vi "Servo Drive Test.vi"() -> ()   [LabVIEW 2019]
uses:
  LINX-PCA9865 PWM/LINX-PCA9865 PWM.lvclass
  LINX-PCA9865 PWM/LINX-PCA9865 PWM.lvclass/LINX-PCA9865 PWM.ctl
  LINX-PCA9865 PWM/Write LINX Resource.vi
  LINX-PCA9865 PWM/Write I2C Slave Address (0x40).vi
  LINX-PCA9865 PWM/Write LINX I2C Channel.vi
  LINX-PCA9865 PWM/Read LINX Resource.vi
  LINX-PCA9865 PWM/Read LINX I2C Channel.vi
  <vilib>/MakerHub/LINX/Public/Utilities/Open Local.vi
  <vilib>/MakerHub/LINX/LMH-LINX.lvlib
panel:
  in  "Slide 2":dbl(slide) scale=-100.0..100.0
  in  "Slide":dbl(slide) scale=-100.0..100.0
  out "New Frequency (Hz)":dbl
  out "Frequency (Hz)":dbl
  in  "stop":bool
  out "Error Out":errorcluster
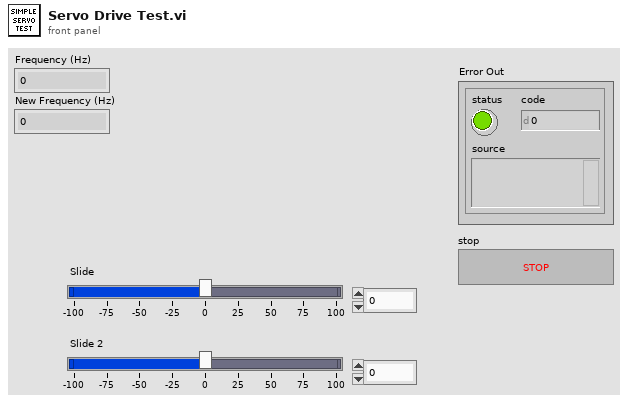
[diagram p1: front panel]
types:
  T1 = typedef "LMH-LINX.lvlib/LINX Ref.ctl" = cluster{"IO":T2, "Interface":T3, "LINX Device Config":T4}
  T2 = typedef "LMH-LINX.lvlib/Platform.ctl" = enum16{"Remote", "Local"}
  T3 = typedef "LMH-LINX.lvlib/Interface.ctl" = enum16{"Serial", "TCP"}
  T4 = typedef "LMH-LINX.lvlib/Device.lvlib/LINX Device Config.ctl" = cluster{"Interface":T3, "COM Port":refnum<visa-resource-name>, "TCP Configuration":T5, "Device Family":u8, "Device ID":u8, "Device Name":string, "TCP Ref":refnum<k5>, "Channels":T6}
  T5 = typedef "LMH-LINX.lvlib/Device.lvlib/TCP Config.ctl" = cluster{"IP Address":string, "Port":u16}
  T6 = typedef "LMH-LINX.lvlib/Channels.ctl" = cluster{"DI":u8[], "DO":u8[], "AI":u8[], "AO":u8[], "PWM":u8[], "QE":u8[], "UART":u8[], "I2C 2":u8[], "SPI":u8[], "CAN":u8[], "Servo":u8[], "AI Ref (V)":dbl, "AI Resolution (Bits)":u8, "AO Ref (V)":dbl, "AO Resolution (Bits)":u8}
  T7 = enum16{"LED/PWM00", "LED/PWM01", "LED/PWM02", "LED/PWM03", "LED/PWM04", "LED/PWM05", "LED/PWM06", "LED/PWM07", "LED/PWM08", "LED/PWM09", "LED/PWM10", "LED/PWM11", "LED/PWM12", "LED/PWM13", "LED/PWM14", "LED/PWM15"}[]
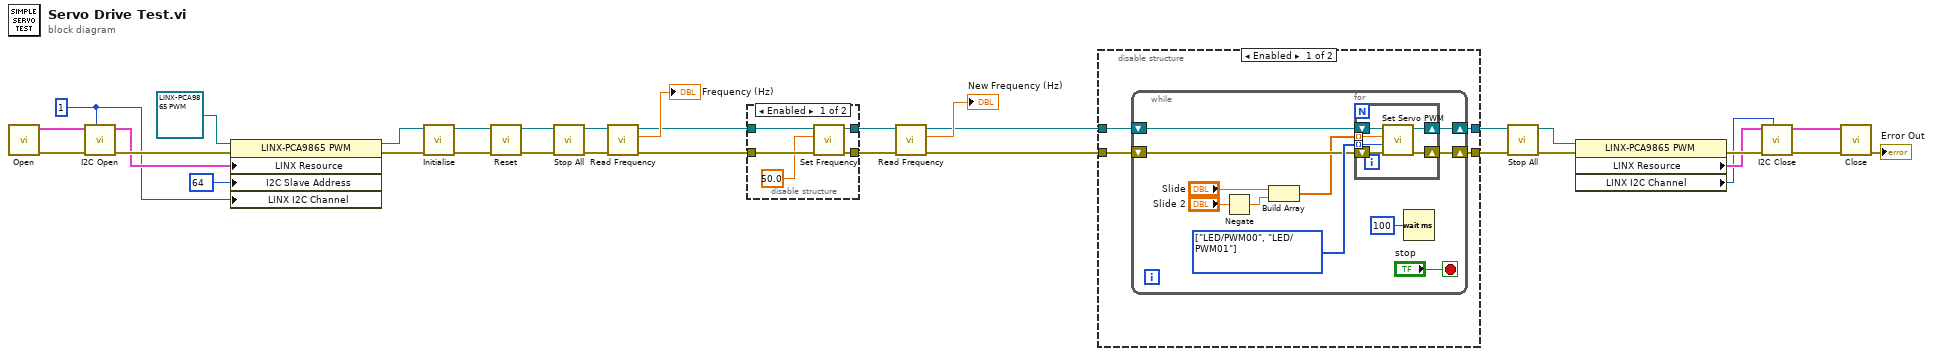
[diagram p0: block diagram]
diagram:
  w24 = u8 1 ("I2C Channel")
  n1 = call-poly <vilib>:"Open.vi"() -> ("Error Out"=w32:errorcluster, "LINX Resource"=w33:T1)  [unwired: 9 in, 1 out]
  n2 = call <vilib>:"I2C Open.vi"("I2C Channel (0)"=w24, "Error In"=w32, "LINX Resource"=w33) -> ("Error Out"=w27:errorcluster, "LINX Resource"=w26:T1)  [unwired: 7 in]
  n3 = property class="LINX-PCA9865 PWM"(reference=refnum<class "LINX-PCA9865 PWM.lvclass"> refnum ("LINX-PCA9865 PWM.lvclass"), error in=w27, "LINX Resource"=w26, "I2C Slave Address"=u8 64 ("I2C Slave Address (0)"), "LINX I2C Channel"=w24) -> (reference out=w22:refnum<class "LINX-PCA9865 PWM.lvclass">, error out=w23:errorcluster)
  n4 = call-dynamic "Initialise.vi"("error in (no error)"=w23, "PWM in"=w22) -> ("error out"=w4:errorcluster, "PWM out"=w5:refnum<class "LINX-PCA9865 PWM.lvclass">)  [unwired: 8 in]
  n5 = call-dynamic "Reset.vi"("error in (no error)"=w4, "PWM in"=w5) -> ("error out"=w3:errorcluster, "PWM out"=w2:refnum<class "LINX-PCA9865 PWM.lvclass">)  [unwired: 8 in]
  n6 = call-dynamic "Stop All.vi"("error in (no error)"=w3, "LINX-PCA9865 PWM in"=w2) -> ("error out"=w14:errorcluster, "LINX-PCA9865 PWM out"=w15:refnum<class "LINX-PCA9865 PWM.lvclass">)  [unwired: 8 in]
  n7 = call-dynamic "Read Frequency.vi"("error in (no error)"=w14, "PWM in"=w15) -> ("error out"=w20:errorcluster, "Frequency (Hz)"=→"Frequency (Hz)":dbl, "PWM out"=w19:refnum<class "LINX-PCA9865 PWM.lvclass">)  [unwired: 7 in]
  n8 = disable-structure shown="Enabled" {
    disable-tunnel: w20 -> [w38 w39]
    disable-tunnel: w19 -> [w37 w40]
    disable-tunnel: [w35 w39] -> w18
    disable-tunnel: [w34 w40] -> w17
    frame Enabled {
      n9 = call-dynamic "Set Frequency.vi"("error in (no error)"=w38, "Frequency (1000Hz)"=50.0, "PWM in"=w37) -> ("error out"=w35:errorcluster, "PWM out"=w34:refnum<class "LINX-PCA9865 PWM.lvclass">)  [unwired: 7 in]
    }
    frame Disabled {
    }
  }
  n10 = call-dynamic "Read Frequency.vi"("error in (no error)"=w18, "PWM in"=w17) -> ("error out"=w11:errorcluster, "Frequency (Hz)"=→"New Frequency (Hz)":dbl, "PWM out"=w12:refnum<class "LINX-PCA9865 PWM.lvclass">)  [unwired: 7 in]
  n11 = disable-structure shown="Enabled" {
    disable-tunnel: w11 -> [w44 w62]
    disable-tunnel: w12 -> [w43 w63]
    disable-tunnel: [w42 w63] -> w10
    disable-tunnel: [w41 w62] -> w13
    frame Enabled {
      n12 = while {
        shift-right: [w52] -> w41
        shift-left: w44 -> [w49]
        shift-right: [w51] -> w42
        shift-left: w43 -> [w53]
        stop <- "stop" stop-if-true
        w50 = T7 [enum."LED/PWM00", enum."LED/PWM01"] items=["LED/PWM00", "LED/PWM01", "LED/PWM02", "LED/PWM03", "LED/PWM04", "LED/PWM05", "LED/PWM06", "LED/PWM07", "LED/PWM08", "LED/PWM09", "LED/PWM10", "LED/PWM11", "LED/PWM12", "LED/PWM13", "LED/PWM14", "LED/PWM15"] ("LEDn (PWM channel)")
        n13 = Negate(x="Slide 2") -> (-x=w46:dbl)
        n14 = Build Array("Slide", w46) -> (w45:dbl[])
        n15 = for {
          tunnel: w45 -> [w58] mode=indexing
          tunnel: w50 -> [w57] mode=indexing
          shift-right: [w59] -> w51
          shift-left: w53 -> [w61]
          shift-right: [w60] -> w52
          shift-left: w49 -> [w56]
          n16 = call "Set Servo PWM.vi"("error in (no error)"=w56, "LEDn (PWM channel)"=w57, "Servo Speed (-100 to 100%)"=w58, "LINX-PCA9865 PWM in"=w61) -> ("error out"=w60:errorcluster, "LINX-PCA9865 PWM out"=w59:refnum<class "LINX-PCA9865 PWM.lvclass">)  [unwired: 6 in]
        }
        n17 = Wait (ms)(milliseconds to wait=u32 100) -> ()  [unwired: 1 out]
      }
    }
    frame Disabled {
    }
  }
  n18 = call-dynamic "Stop All.vi"("error in (no error)"=w13, "LINX-PCA9865 PWM in"=w10) -> ("error out"=w8:errorcluster, "LINX-PCA9865 PWM out"=w9:refnum<class "LINX-PCA9865 PWM.lvclass">)  [unwired: 8 in]
  n19 = property class="LINX-PCA9865 PWM"(reference=w9, error in=w8) -> (error out=w7:errorcluster, "LINX Resource"=w6:T1, "LINX I2C Channel"=w1:u8)  [unwired: 1 out]
  n20 = call <vilib>:"I2C Close.vi"("I2C Channel (0)"=w1, "Error In"=w7, "LINX Resource"=w6) -> ("Error Out"=w31:errorcluster, "LINX Resource"=w30:T1)  [unwired: 7 in]
  n21 = call <vilib>:"Close.vi"("Error In"=w31, "LINX Resource"=w30) -> ("Error Out"=→"Error Out":errorcluster)  [unwired: 9 in]
